vi "SimulatedConfigRefGlobal.vi"() -> ()   [LabVIEW 2017, in "ScanEngine.lvlib"]
uses:
  <vilib>/addons/InsightCM/Devices/Shared/Common/ScanEngine/ScanEngine.lvlib
  <vilib>/addons/InsightCM/Devices/Shared/Common/ScanEngine/controls/SimConfigRefs.ctl
panel:
  in  "Simulated Config Refs":T1
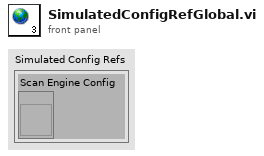
[diagram p1: front panel]
types:
  T1 = typedef "ScanEngine.lvlib/SimConfigRefs.ctl" = cluster{"Scan Engine Config":refnum<vi>}
diagram:
